vi "Class Implements Method.vi"(8 "error in (no error)":errorcluster, 10 "Method Name":string, 11 "Class Refnum":refnum<vi>) -> (0 "error out":errorcluster, 1 "VI Qualified Name":string, 2 "Implements method?":bool, 3 "Class Refnum out":refnum<vi>)   [LabVIEW 2020, in "Peek Window.lvlib"]
uses:
  Peek Window.lvlib
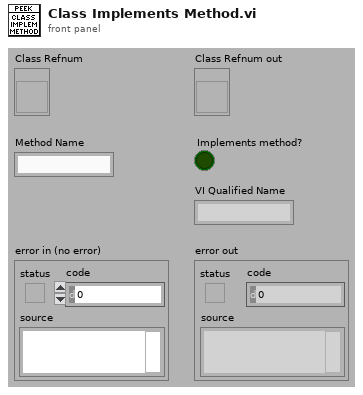
[diagram p1: front panel]
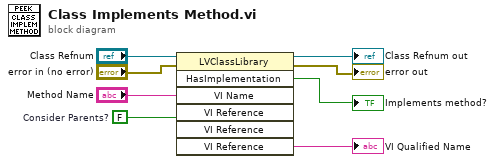
[diagram p0: block diagram]
diagram:
  w1 = FALSE  # Consider Parents?
  n1 = invoke class="LVClassLibrary" method="HasImplementation"(reference="Class Refnum", error in="error in (no error)", "VI Name"="Method Name", "VI Reference"=w1) -> (reference out=→"Class Refnum out":refnum<vi>, error out=→"error out":errorcluster, "HasImplementation"=→"Implements method?":bool, "VI Reference"=→"VI Qualified Name":string)  [unwired: 3 in, 3 out]
